vi "Copy Firmware Libraries.vi"(8 "Error In":errorcluster, 11 "Library Destination Dir":path=path "C:/Program Files (x86)/National Instruments/LabVIEW 2011/vi.lib/LabVIEW Hacker/LINX/Firmware/Source/librariestest") -> (0 "Error Out":errorcluster)   [LabVIEW 2020, in "LMH-LINX.lvlib"]
uses:
  LMH-LINX.lvlib
  Type Defs/Firmware Library Component.ctl
  <vilib>/Utility/config.llb/Read Key (String).vi
  <vilib>/Utility/config.llb/NI_LVConfig.lvlib
  Toolbox/LMH-Toolbox.lvlib
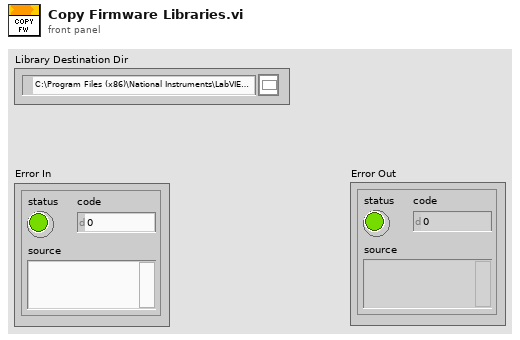
[diagram p1: front panel]
types:
  T1 = typedef "NI_LVConfig.lvlib/Config Data RefNum.ctl" = refnum<k1>
  T2 = typedef "LMH-LINX.lvlib/Firmware Library Component.ctl" = cluster{"Source":path, "Destination":path}
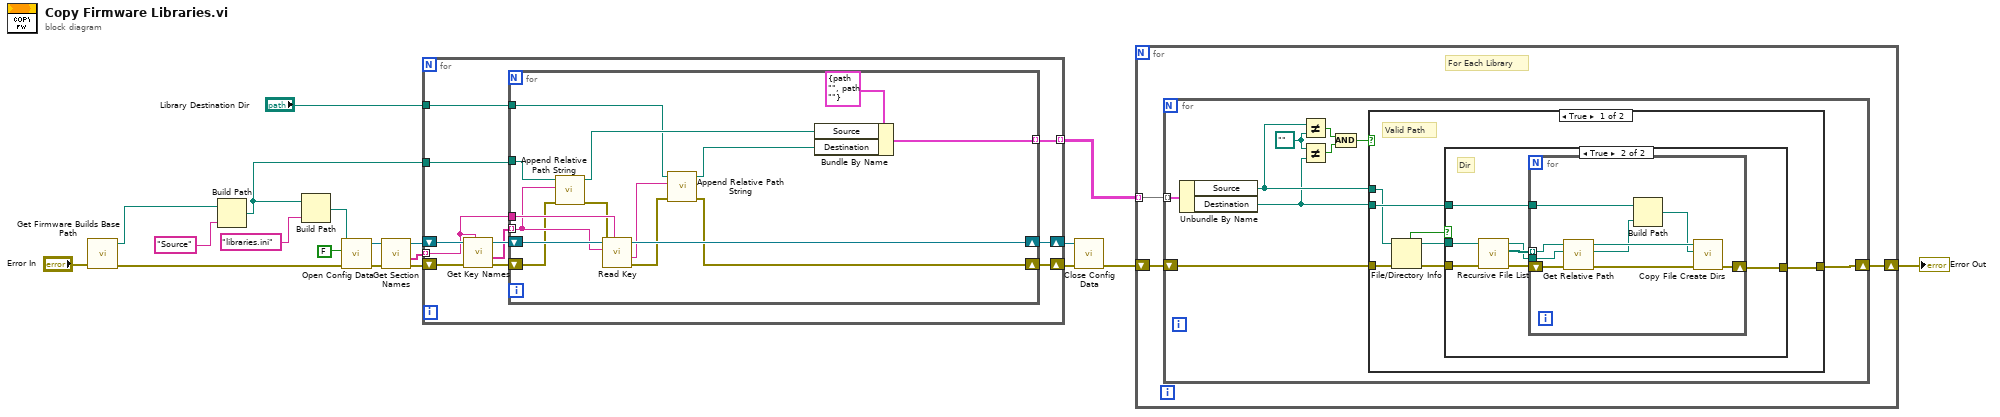
[diagram p0: block diagram]
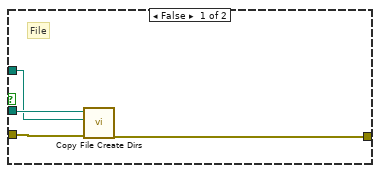
[diagram p2: hidden frame]
diagram:
  n1 = call "Get Firmware Builds Base Path.vi"("Error In"="Error In") -> ("Error Out"=w2:errorcluster, "Firmware Builds Base Path"=w1:path)  [unwired: 9 in]
  n2 = Build Path(base path=w1, name or relative path="Source") -> (appended path=w3:path)
  n3 = Build Path(base path=w3, name or relative path="libraries.ini") -> (appended path=w7:path)
  n4 = call <vilib>:"Open Config Data.vi"("error in (no error)"=w2, "create file if necessary (T)"=FALSE, "configuration file path"=w7) -> ("error out"=w18:errorcluster, "refnum"=w19:T1)  [unwired: 6 in, 1 out]
  n5 = call <vilib>:"Get Section Names.vi"("error in (no error)"=w18, "refnum"=w19) -> ("error out"=w14:errorcluster, "section names"=w12:string[], "refnum out"=w16:T1)  [unwired: 7 in]
  n6 = for {
    shift-right: [w27] -> w15
    shift-left: w16 -> [w30]
    shift-right: [w25] -> w13
    shift-left: w14 -> [w29]
    tunnel: w12 -> [w23] mode=indexing
    tunnel: w3 -> [w22]
    tunnel: [w21] -> w11 mode=indexing
    tunnel: "Library Destination Dir" -> [w20]
    n7 = call <vilib>:"Get Key Names.vi"("section"=w23, "error in (no error)"=w29, "refnum"=w30) -> ("error out"=w26:errorcluster, "key names"=w24:string[], "refnum out"=w28:T1)  [unwired: 5 in, 1 out]
    n8 = for {
      shift-right: [w44] -> w27
      shift-left: w28 -> [w45]
      shift-right: [w35] -> w25
      shift-left: w26 -> [w37]
      tunnel: w24 -> [w38] mode=indexing
      tunnel: w23 -> [w43]
      tunnel: w22 -> [w39]
      tunnel: [w32] -> w21 mode=indexing
      tunnel: w20 -> [w31]
      n9 = call "Append Relative Path String.vi"("Error In"=w37, "Relative Path"=w38, "Base Path"=w39) -> ("Error Out"=w36:errorcluster, "Absolute Path"=w34:path)  [unwired: 7 in]
      n10 = call-poly <vilib>:"Read Key.vi"("section"=w43, "error in (no error)"=w36, "key"=w38, "refnum"=w45) -> ("error out"=w42:errorcluster, "value"=w41:string, "refnum out"=w44:T1)  [unwired: 4 in, 1 out]
      n11 = call "Append Relative Path String.vi"("Error In"=w42, "Relative Path"=w41, "Base Path"=w31) -> ("Error Out"=w35:errorcluster, "Absolute Path"=w33:path)  [unwired: 7 in]
      n12 = Bundle By Name(cluster=T2 {"Source"=path "", "Destination"=path ""} ("Library Component"), "Source"=w34, "Destination"=w33) -> (w32:T2)
    }
  }
  n13 = call <vilib>:"Close Config Data.vi"("error in (no error)"=w13, "refnum"=w15) -> ("error out"=w10:errorcluster)  [unwired: 8 in, 1 out]
  n14 = for {
    tunnel: w11 -> [w47] mode=indexing
    shift-right: [w46] -> w9
    shift-left: w10 -> [w48]
    # "For Each Library"
    n15 = for {
      tunnel: w47 -> [w57] mode=indexing
      shift-right: [w56] -> w46
      shift-left: w48 -> [w49]
      w53 = path ""
      n16 = Unbundle By Name(w57) -> ("Source"=w52:path, "Destination"=w51:path)
      n17 = Not Equal?(x=w52, y=w53) -> (x != y?=w55:bool)
      n18 = Not Equal?(x=w53, y=w51) -> (x != y?=w54:bool)
      n19 = And(x=w55, y=w54) -> (x .and. y?=w50:bool)
      n20 = case shown="True" w50 {
        tunnel: [w63 w85] -> w56
        tunnel: w51 -> [w64 _]
        tunnel: w52 -> [w61 _]
        tunnel: w49 -> [w62 w85]
        frame True {
          # "Valid Path"
          n21 = File/Directory Info(path=w61, error in=w62) -> (path out=w60:path, directory=w58:bool, error out=w59:errorcluster)  [unwired: 4 out]
          n22 = case shown="True" w58 {
            tunnel: w64 -> [w66 w72]
            tunnel: [w65 w71] -> w63
            tunnel: w60 -> [w67 w70]
            tunnel: w59 -> [w68 w69]
            frame False {
              # "File"
              n23 = call "Copy File Create Dirs.vi"("Error In"=w68, "Destination"=w66, "Source"=w67) -> ("Error Out"=w65:errorcluster)  [unwired: 8 in]
            }
            frame True {
              # "Dir"
              n24 = call <vilib>:"Recursive File List.vi"("error in (no error)"=w69, "Folder Path"=w70) -> ("error out"=w75:errorcluster, "All Files in Dir"=w74:path[], "dup Folder Path"=w73:path)  [unwired: 5 in, 2 out]
              n25 = for {
                tunnel: w74 -> [w83] mode=indexing
                tunnel: w73 -> [w82]
                tunnel: w72 -> [w79]
                shift-right: [w76] -> w71
                shift-left: w75 -> [w84]
                n26 = call "Get Relative Path.vi"("Error In"=w84, "Relative Path Root"=w82, "File / Folder"=w83) -> ("Error Out"=w81:errorcluster, "Relative Path"=w78:path, "Duplicate File / Folder"=w80:path)  [unwired: 6 in]
                n27 = Build Path(base path=w79, name or relative path=w78) -> (appended path=w77:path)
                n28 = call "Copy File Create Dirs.vi"("Error In"=w81, "Destination"=w77, "Source"=w80) -> ("Error Out"=w76:errorcluster)  [unwired: 8 in]
              }
            }
          }
        }
        frame False {
          # "Invalid Path"
        }
      }
    }
  }
  "Error Out" <- w9
